vi "Get Auton Command VI.vi"(1 "Autonomous Command Name":T1) -> (0 "VI Refnum":refnum<vi>)   [LabVIEW 2016]
uses:
  Autonomous Commands/Autonomous Command Names.ctl
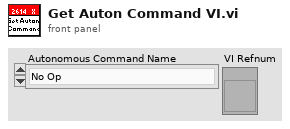
[diagram p1: front panel]
types:
  T1 = typedef "Autonomous Command Names.ctl" = enum16{"No Op", "Command Drive+Climb Shift", "Command Wait", "Command Deliver Gear", "Command Buffer", "Command Drive Path", "Command Drive Time", "Command Shoot", "Command Turn to Heading", "Command Run Conveyor", "Command Spinup Shooter", "Command Deliver Gear Front", "Command Toggle Intake Rotation", "DO NOT USE", "Command Agitate Hopper", "Command Pre-Buffer", "Command Turn to Target", "Command Deliver Gear with Safety", "Command Drive Time with IMU", "Command Drive to Encoders"}
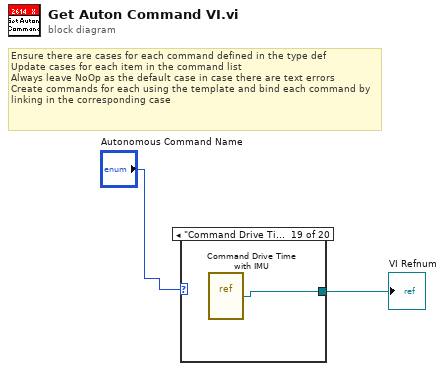
[diagram p0: block diagram]
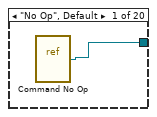
[diagram p2: hidden frame]
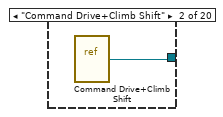
[diagram p3: hidden frame]
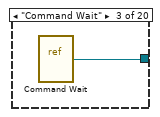
[diagram p4: hidden frame]
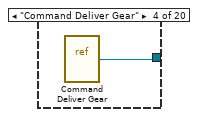
[diagram p5: hidden frame]
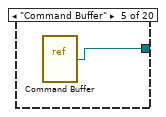
[diagram p6: hidden frame]
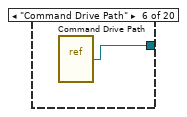
[diagram p7: hidden frame]
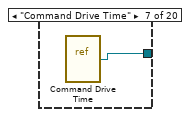
[diagram p8: hidden frame]
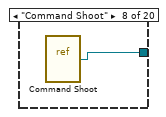
[diagram p9: hidden frame]
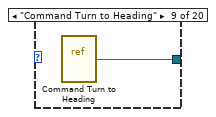
[diagram p10: hidden frame]
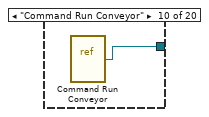
[diagram p11: hidden frame]
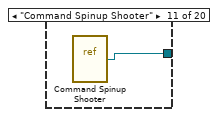
[diagram p12: hidden frame]
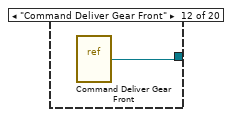
[diagram p13: hidden frame]
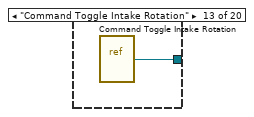
[diagram p14: hidden frame]
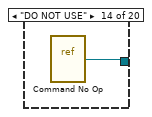
[diagram p15: hidden frame]
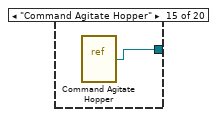
[diagram p16: hidden frame]
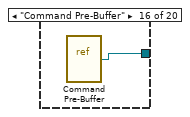
[diagram p17: hidden frame]
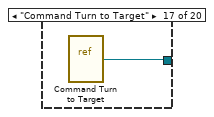
[diagram p18: hidden frame]
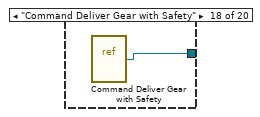
[diagram p19: hidden frame]
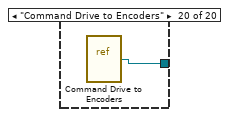
[diagram p20: hidden frame]
diagram:
  # "Ensure there are cases for each command defined in the type def\nUpdate cases for each item in the command list\nAlways leave NoOp as the default case in case there are text errors\nCreate commands for each using the template and bind each command by linking in the corresponding case"
  n1 = case shown="\"Command Drive Time with IMU\"" "Autonomous Command Name" {
    tunnel: [w3 w4 w5 w6 w7 w8 w9 w10 w11 w12 w13 w14 w15 w16 w17 w18 w19 w20 w21 w22] -> w1
    frame "No Op", Default {
      n2 = vi-ref "Command No Op.vi"() -> (w3:refnum<vi>)
    }
    frame "Command Drive+Climb Shift" {
      n3 = vi-ref "Command Drive+Climb Shift.vi"() -> (w4:refnum<vi>)
    }
    frame "Command Wait" {
      n4 = vi-ref "Command Wait.vi"() -> (w5:refnum<vi>)
    }
    frame "Command Deliver Gear" {
      n5 = vi-ref "Command Deliver Gear.vi"() -> (w6:refnum<vi>)
    }
    frame "Command Buffer" {
      n6 = vi-ref "Command Buffer.vi"() -> (w7:refnum<vi>)
    }
    frame "Command Drive Path" {
      n7 = vi-ref "Command Drive Path.vi"() -> (w8:refnum<vi>)
    }
    frame "Command Drive Time" {
      n8 = vi-ref "Command Drive Time.vi"() -> (w9:refnum<vi>)
    }
    frame "Command Shoot" {
      n9 = vi-ref "Command Shoot.vi"() -> (w10:refnum<vi>)
    }
    frame "Command Turn to Heading" {
      n10 = vi-ref "Command Turn to Heading.vi"() -> (w11:refnum<vi>)
    }
    frame "Command Run Conveyor" {
      n11 = vi-ref "Command Run Conveyor.vi"() -> (w12:refnum<vi>)
    }
    frame "Command Spinup Shooter" {
      n12 = vi-ref "Command Spinup Shooter.vi"() -> (w13:refnum<vi>)
    }
    frame "Command Deliver Gear Front" {
      n13 = vi-ref "Command Deliver Gear Front.vi"() -> (w14:refnum<vi>)
    }
    frame "Command Toggle Intake Rotation" {
      n14 = vi-ref "Command Toggle Intake Rotation.vi"() -> (w15:refnum<vi>)
    }
    frame "DO NOT USE" {
      n15 = vi-ref "Command No Op.vi"() -> (w16:refnum<vi>)
    }
    frame "Command Agitate Hopper" {
      n16 = vi-ref "Command Agitate Hopper.vi"() -> (w17:refnum<vi>)
    }
    frame "Command Pre-Buffer" {
      n17 = vi-ref "Command Pre-Buffer.vi"() -> (w18:refnum<vi>)
    }
    frame "Command Turn to Target" {
      n18 = vi-ref "Command Turn to Target.vi"() -> (w19:refnum<vi>)
    }
    frame "Command Deliver Gear with Safety" {
      n19 = vi-ref "Command Deliver Gear with Safety.vi"() -> (w20:refnum<vi>)
    }
    frame "Command Drive Time with IMU" {
      n20 = vi-ref "Command Drive Time with IMU.vi"() -> (w21:refnum<vi>)
    }
    frame "Command Drive to Encoders" {
      n21 = vi-ref "Command Drive to Encoders.vi"() -> (w22:refnum<vi>)
    }
  }
  "VI Refnum" <- w1
